vi "AIT 1553 - Parse Tree Messages.vi"(5 "FIFO Idx Qs":T10, 6 "Bus Config Info":T2, 7 "Bus Section":T1, 8 "error out":errorcluster, 10 "Message Refs":T11[](array[typedef]) format="%.0x", 11 "Custom Device Ref":T11 format="%.0x") -> (0 "error out":errorcluster, 2 "Msg Names":string[](array[string]), 3 "Message Settings":T4[](array[typedef]) {"Driver Data"."First Word" min=8 max=31; "Driver Data"."Num Bits" min=1 max=32; "Driver Data"."Start Bit" min=8 max=31; "Block Data Refs"."Data Reference" format="%.0x"})   [LabVIEW 2013, in "AIT 1553 Custom Device.lvlib"]
uses:
  AIT 1553 Custom Device.lvlib
  <vilib>/NI Veristand/Custom Device API/Custom Device Item Ref.ctl
  RT Controls/FIFO Idx Qs.ctl
  RT Controls/AIT 1553 - RT Message Settings.ctl
  <vilib>/NI Veristand/Custom Device API/Block Data Reference.ctl
  <vilib>/NI Veristand/Custom Device API/Data Reference.ctl
  RT Controls/AIT 1553 - Driver Data.ctl
  Controls and Global/Start Bit.ctl
  Controls and Global/Number of Bits.ctl
  RT Controls/AIT 1553 - Board Config Info.ctl
  RT Controls/AIT 1553 - Hardware Type.ctl
  RT Controls/AIT 1553 - Bus Section.ctl
  <vilib>/NI Veristand/Custom Device Tools/Custom Device Utility Library/RT Debug String Color Spec.ctl
  RT Controls/Data Ref FGV Command.ctl
  <instrlib>/AIT 1553/Public/AIT 1553 Controls/Xfer Direction.ctl
  <vilib>/NI Veristand/Custom Device API/Data Access Type.ctl
  Controls and Global/Global.vi
  <vilib>/NI Veristand/Custom Device API/Get Item Property (I32).vi
  <vilib>/NI Veristand/Custom Device API/Get Item Property (Double Array).vi
  <vilib>/NI Veristand/Custom Device API/Get Item Property (U32).vi
  <vilib>/NI Veristand/Custom Device API/Get Item Property (Boolean).vi
  <vilib>/NI Veristand/Custom Device Tools/Custom Device Utility Library/NI VeriStand - Search for Item.vi
  <vilib>/NI Veristand/Custom Device Tools/Custom Device Utility Library/NI VeriStand - Search for All Items by GUID.vi
  <vilib>/NI Veristand/Custom Device Tools/Custom Device Utility Library/NI VeriStand - Search for Item by GUID.vi
  Utility/Print NIVS Debug String.vi
  <vilib>/NI Veristand/Custom Device API/Get Item Property (Double).vi
  <vilib>/NI Veristand/Custom Device API/Custom Device API.lvlib
  <instrlib>/AIT 1553/AIT 1553.lvlib
  <vilib>/NI Veristand/Custom Device Tools/Custom Device Utility Library/Custom Device Utility Library.lvlib
panel:
  in  "Channel handle in":u32
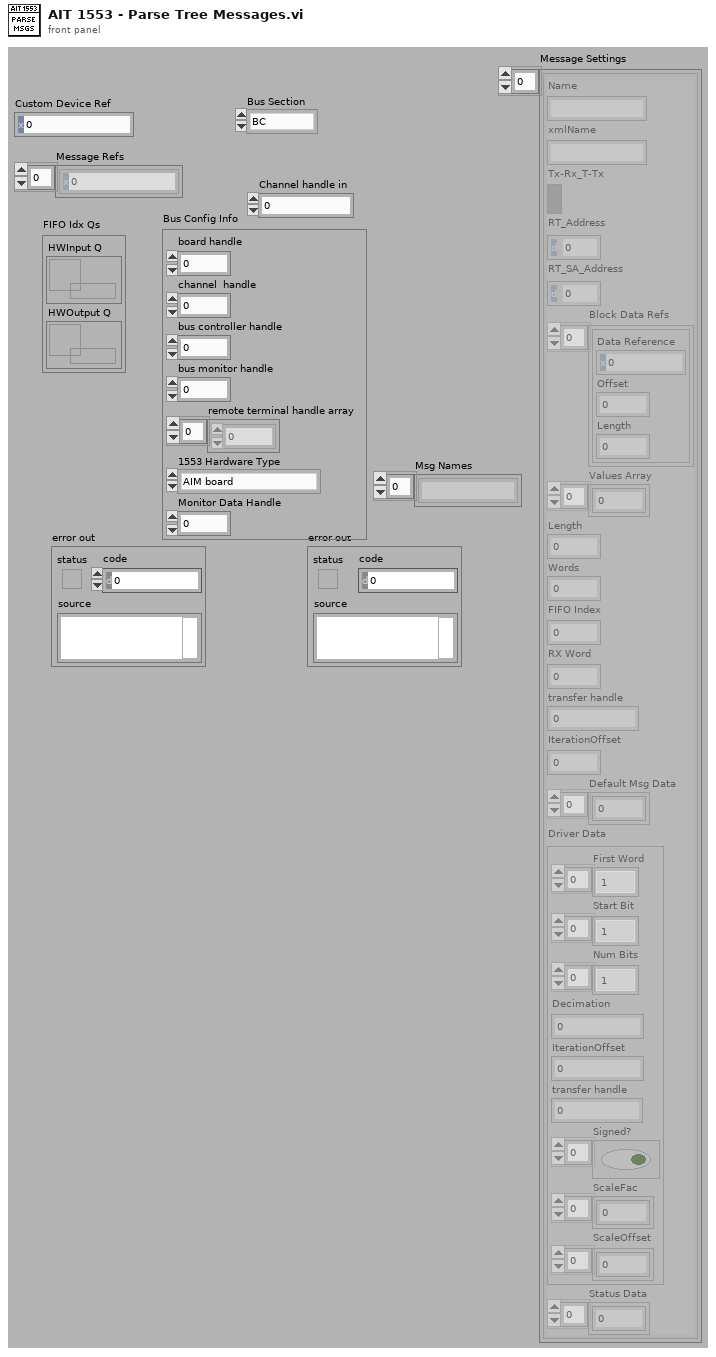
[diagram p1: front panel]
types:
  T1 = typedef "AIT 1553 Custom Device.lvlib/AIT 1553 - Bus Section.ctl" = enum16{"BC", "BM", "RT"}
  T2 = typedef "AIT 1553 Custom Device.lvlib/AIT 1553 - Board Config Info.ctl" = cluster{"board handle":u32, "channel  handle":u32, "bus controller handle":u32, "bus monitor handle":u32, "remote terminal handle array":u32[], "1553 Hardware Type":T3, "Monitor Data Handle":u32}
  T3 = typedef "AIT 1553 Custom Device.lvlib/AIT 1553 - Hardware Type.ctl" = enum16{"AIM board", "AIT Board"}
  T4 = typedef "AIT 1553 Custom Device.lvlib/AIT 1553 - RT Message Settings.ctl" = cluster{"Name":string, "xmlName":string, "Tx-Rx_T-Tx":bool, "RT_Address":u8, "RT_SA_Address":u8, "Block Data Refs":T5[], "Values Array":dbl[], "Length":i32, "Words":i32, "FIFO Index":i32, "RX Word":u32, "transfer handle":u32, "IterationOffset":i32, "Default Msg Data":u16[], "Driver Data":T7, "Status Data":u32[]}
  T5 = typedef "Custom Device API.lvlib/Block Data Reference.ctl" = cluster{"Data Reference":T6, "Offset":i32, "Length":i32}
  T6 = typedef "Custom Device API.lvlib/Data Reference.ctl" = i32
  T7 = typedef "AIT 1553 Custom Device.lvlib/AIT 1553 - Driver Data.ctl" = cluster{"First Word":T8[], "Start Bit":T8[], "Num Bits":T9[], "Decimation":i32, "IterationOffset":i32, "transfer handle":u32, "Signed?":bool[], "ScaleFac":dbl[], "ScaleOffset":dbl[]}
  T8 = typedef "AIT 1553 Custom Device.lvlib/Start Bit.ctl" = i32
  T9 = typedef "AIT 1553 Custom Device.lvlib/Number of Bits.ctl" = i32
  T10 = typedef "AIT 1553 Custom Device.lvlib/FIFO Idx Qs.ctl" = cluster{"HWInput Q":refnum<queue>, "HWOutput Q":refnum<queue>}
  T11 = typedef "Custom Device API.lvlib/Custom Device Item Ref.ctl" = u64
  T12 = typedef "Custom Device Utility Library.lvlib/RT Debug String Color Spec.ctl" = u16
  T13 = typedef "AIT 1553.lvlib/Xfer Direction.ctl" = enum16{"RECEIVE_TRANSFER", "TRANSMIT_TRANSFER"}
  T14 = typedef "AIT 1553 Custom Device.lvlib/Data Ref FGV Command.ctl" = enum16{"Intialize", "Get", "Update"}
  T15 = typedef "Custom Device API.lvlib/Data Access Type.ctl" = enum16{"Read", "Write"}
  T16 = typedef "Custom Device API.lvlib/Custom Device Item Info.ctl" = cluster{"Name":string, "Is Channel":bool, "GUID":string, "Is Waveform":bool}
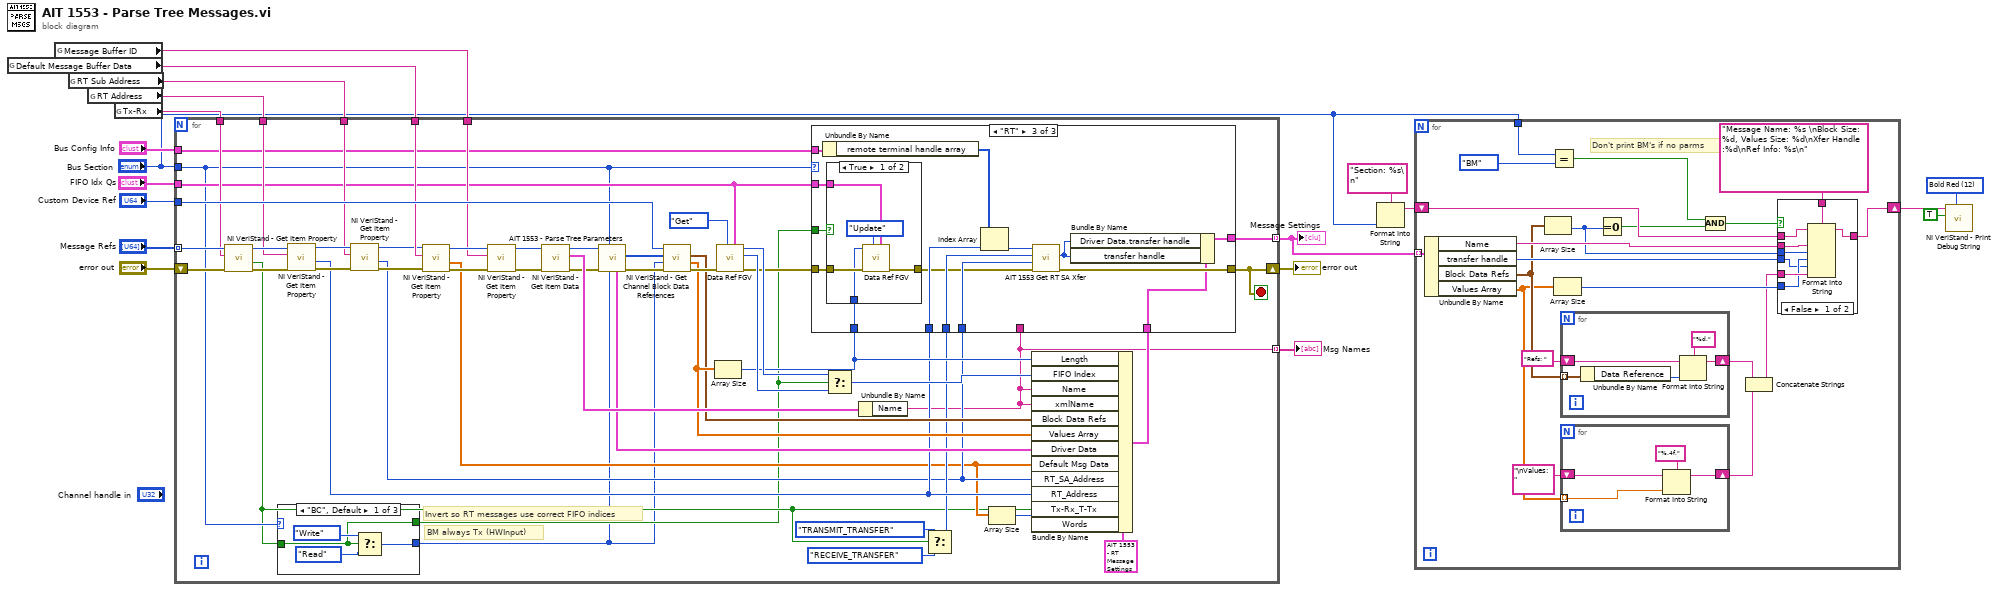
[diagram p0: block diagram]
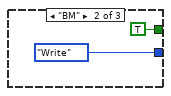
[diagram p3: hidden frame]
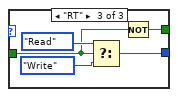
[diagram p4: hidden frame]
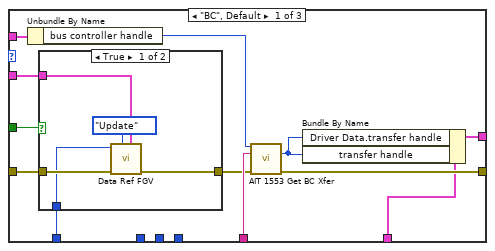
[diagram p5: hidden frame]
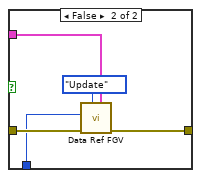
[diagram p6: hidden frame]
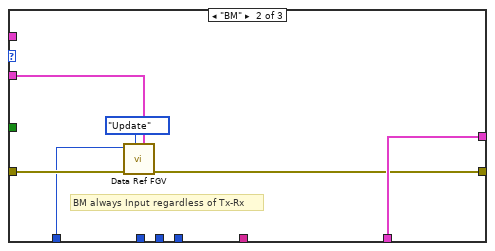
[diagram p7: hidden frame]
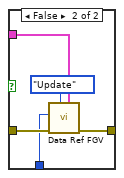
[diagram p8: hidden frame]
diagram:
  w1 = T12 12 items=["Plain White"=7, "Bold White"=15, "Bold Blue"=9, "Bold Green"=10, "Bold Red"=12] ("Attribute")
  n1 = global read "Global.vi" "Default Message Buffer Data"() -> (w11:string)
  n2 = global read "Global.vi" "Message Buffer ID"() -> (w10:string)
  n3 = global read "Global.vi" "RT Sub Address"() -> (w12:string)
  n4 = global read "Global.vi" "RT Address"() -> (w13:string)
  n5 = global read "Global.vi" "Tx-Rx"() -> (w14:string)
  n6 = for {
    tunnel: "Message Refs" -> [w70] mode=indexing
    shift-right: [w60] -> w16
    shift-left: "error out" -> [w61]
    tunnel: "Custom Device Ref" -> [w59]
    tunnel: "FIFO Idx Qs" -> [w33]
    tunnel: w14 -> [w58]
    tunnel: w11 -> [w57]
    tunnel: w13 -> [w52]
    tunnel: w12 -> [w47]
    tunnel: w10 -> [w42]
    tunnel: [w34] -> w4 mode=indexing
    tunnel: "Bus Section" -> [w26]
    tunnel: "Bus Config Info" -> [w32]
    tunnel: [w25] -> w8 mode=indexing
    stop <- w60 stop-if-true
    # "BM always Tx (HWInput)"
    # "Invert so RT messages use correct FIFO indices"
    n7 = call-poly <vilib>:"NI VeriStand - Get Item Property.vi"("error in (no error)"=w61, "Property Name"=w58, "Item Ref in"=w70) -> ("error out"=w53:errorcluster, "Value"=w22:bool, "Item Ref out"=w54:T11)  [unwired: 5 in, 1 out]
    n8 = case shown="\"BC\", Default" w26 {
      tunnel: [w72 Data_Access_Type."Write" ("y") w79] -> w20
      tunnel: w22 -> [w71 _ w78]
      tunnel: [w71 TRUE ("Value") w77] -> w21
      frame "BC", Default {
        n9 = Select(t=Data_Access_Type."Write" ("y"), s=w71, f=Data_Access_Type."Read" ("y")) -> (s? t:f=w72:T15)
      }
      frame "BM" {
      }
      frame "RT" {
        n10 = Select(t=Data_Access_Type."Read" ("y"), s=w78, f=Data_Access_Type."Write" ("y")) -> (s? t:f=w79:T15)
        n11 = Not(x=w78) -> (.not. x?=w77:bool)
      }
    }
    n12 = call-poly <vilib>:"NI VeriStand - Get Item Property.vi"("error in (no error)"=w53, "Property Name"=w52, "Item Ref in"=w54) -> ("error out"=w49:errorcluster, "Value"=w31:i32, "Item Ref out"=w51:T11)  [unwired: 5 in, 1 out]
    n13 = call-poly <vilib>:"NI VeriStand - Get Item Property.vi"("error in (no error)"=w49, "Property Name"=w47, "Item Ref in"=w51) -> ("error out"=w48:errorcluster, "Value"=w27:u32, "Item Ref out"=w50:T11)  [unwired: 5 in, 1 out]
    n14 = call-poly <vilib>:"NI VeriStand - Get Item Property.vi"("error in (no error)"=w48, "Property Name"=w57, "Item Ref in"=w50) -> ("error out"=w44:errorcluster, "Value"=w24:dbl[], "Item Ref out"=w46:T11)  [unwired: 5 in, 1 out]
    n15 = call-poly <vilib>:"NI VeriStand - Get Item Property.vi"("error in (no error)"=w44, "Property Name"=w42, "Item Ref in"=w46) -> ("error out"=w43:errorcluster, "Item Ref out"=w45:T11)  [unwired: 5 in, 2 out]
    n16 = call <vilib>:"NI VeriStand - Get Item Data.vi"("error in (no error)"=w43, "Item Ref in"=w45) -> ("error out"=w56:errorcluster, "Item Info"=w69:T16, "Item Ref out"=w55:T11)  [unwired: 6 in, 1 out]
    n17 = call "AIT 1553 - Parse Tree Parameters.vi"("Access Type"=w20, "Bus Section"=w26, "error in"=w56, "Item Ref in"=w55) -> ("error out"=w67:errorcluster, "Parameter References"=w68:T11[], "Parameter Driver Data"=w38:T7)  [unwired: 4 in, 1 out]
    n18 = call <vilib>:"NI VeriStand - Get Channel Block Data References.vi"("error in (no error)"=w67, "Access"=w20, "Channel Refs"=w68, "Device Ref in"=w59) -> ("error out"=w66:errorcluster, "Values Array"=w40:dbl[], "Block Data Refs"=w39:T5[])  [unwired: 4 in, 1 out]
    n19 = Array Size(array=w40) -> (size(s)=w37:i32)
    n20 = call "Data Ref FGV.vi"("FIFO Idx Qs"=w33, "Command"=Data_Ref_FGV_Command."Get", "error in (no error)"=w66) -> ("error out"=w62:errorcluster, "HWOutput FIFO Index / Length"=w63:i32, "HWInput FIFO Index / Length"=w64:i32)  [unwired: 6 in]
    n21 = Select(t=w64, s=w21, f=w63) -> (s? t:f=w36:i32)
    n22 = Unbundle By Name(w69) -> ("Name"=w25:string)
    n23 = Select(t=Xfer_Direction."TRANSMIT_TRANSFER" ("direction in"), s=w22, f=Xfer_Direction."RECEIVE_TRANSFER" ("direction in")) -> (s? t:f=w28:T13)
    n24 = Array Size(array=w24) -> (size(s)=w23:i32)
    n25 = Bundle By Name(cluster=T4 {"Name"="", "xmlName"="", "Tx-Rx_T-Tx"=FALSE, "RT_Address"=0, "RT_SA_Address"=0, "Block Data Refs"=[], "Values Array"=[], "Length"=0, "Words"=0, "FIFO Index"=0, "RX Word"=0, "transfer handle"=0, "IterationOffset"=0, "Default Msg Data"=[], "Driver Data"={"First Word"=[], "Start Bit"=[], "Num Bits"=[], "Decimation"=0, "IterationOffset"=0, "transfer handle"=0, "Signed?"=[], "ScaleFac"=[], "ScaleOffset"=[]}, "Status Data"=[]} ("Message Settings"), "Length"=w37, "FIFO Index"=w36, "Name"=w25, "xmlName"=w25, "Block Data Refs"=w39, "Values Array"=w40, "Driver Data"=w38, "Default Msg Data"=w24, "RT_SA_Address"=w27, "RT_Address"=w31, "Tx-Rx_T-Tx"=w22, "Words"=w23) -> (w35:T4)
    n26 = case shown="\"RT\"" w26 {
      tunnel: w62 -> [w93 w108 w114]
      tunnel: [w85 w104 w123] -> w60
      tunnel: w37 -> [w92 w106 w112]
      tunnel: w35 -> [w84 w105 w122]
      tunnel: [w83 w105 w121] -> w34
      tunnel: w25 -> [w88 _ _]
      tunnel: w21 -> [w91 _ w115]
      tunnel: w33 -> [w90 w107 w111]
      tunnel: w32 -> [w89 _ w124]
      tunnel: w31 -> [_ _ w120]
      tunnel: w28 -> [_ _ w119]
      tunnel: w27 -> [_ _ w118]
      frame "BC", Default {
        n27 = Unbundle By Name(w89) -> ("bus controller handle"=w87:u32)
        n28 = case shown="True" w91 {
          tunnel: w93 -> [w98 w103]
          tunnel: w92 -> [w96 w101]
          tunnel: w90 -> [w95 w100]
          tunnel: [w94 w99] -> w86
          frame True {
            n29 = call "Data Ref FGV.vi"("FIFO Idx Qs"=w95, "Command"=Data_Ref_FGV_Command."Update", "error in (no error)"=w98, "HWInput Length"=w96) -> ("error out"=w94:errorcluster)  [unwired: 5 in, 2 out]
          }
          frame False {
            n30 = call "Data Ref FGV.vi"("FIFO Idx Qs"=w100, "Command"=Data_Ref_FGV_Command."Update", "error in (no error)"=w103, "HWOutput Length"=w101) -> ("error out"=w99:errorcluster)  [unwired: 5 in, 2 out]
          }
        }
        n31 = call <instrlib>:"AIT 1553 Get BC Xfer.vi"("bus controller handle in"=w87, "transfer description"=w88, "error in"=w86) -> ("transfer handle out"=w82:u32, "error out"=w85:errorcluster)  [unwired: 10 in, 1 out]
        n32 = Bundle By Name(cluster=w84, "Driver Data.transfer handle"=w82, "transfer handle"=w82) -> (w83:T4)
      }
      frame "BM" {
        # "BM always Input regardless of Tx-Rx"
        n33 = call "Data Ref FGV.vi"("FIFO Idx Qs"=w107, "Command"=Data_Ref_FGV_Command."Update", "error in (no error)"=w108, "HWInput Length"=w106) -> ("error out"=w104:errorcluster)  [unwired: 5 in, 2 out]
      }
      frame "RT" {
        n34 = Unbundle By Name(w124) -> ("remote terminal handle array"=w116:u32[])
        n35 = case shown="True" w115 {
          tunnel: w114 -> [w129 w134]
          tunnel: [w127 w131] -> w113
          tunnel: w112 -> [w125 w130]
          tunnel: w111 -> [w126 w132]
          frame True {
            n36 = call "Data Ref FGV.vi"("FIFO Idx Qs"=w126, "Command"=Data_Ref_FGV_Command."Update", "error in (no error)"=w129, "HWInput Length"=w125) -> ("error out"=w127:errorcluster)  [unwired: 5 in, 2 out]
          }
          frame False {
            n37 = call "Data Ref FGV.vi"("FIFO Idx Qs"=w132, "Command"=Data_Ref_FGV_Command."Update", "error in (no error)"=w134, "HWOutput Length"=w130) -> ("error out"=w131:errorcluster)  [unwired: 5 in, 2 out]
          }
        }
        n38 = Index Array(array=w116, index=w120) -> (element=w117:u32)
        n39 = call <instrlib>:"AIT 1553 Get RT SA Xfer.vi"("error in"=w113, "subaddress in"=w118, "direction in"=w119, "remote terminal handle in"=w117) -> ("error out"=w123:errorcluster, "transfer handle out"=w110:u32)  [unwired: 5 in, 1 out]
        n40 = Bundle By Name(cluster=w122, "Driver Data.transfer handle"=w110, "transfer handle"=w110) -> (w121:T4)
      }
    }
  }
  "error out" <- w16
  "Message Settings" <- w4
  "Msg Names" <- w8
  n41 = Format Into String(format string="Section: %s\n", "Bus Section") -> (resulting string=w7:string)  [unwired: 2 in, 1 out]
  n42 = for {
    tunnel: w4 -> [w154] mode=indexing
    shift-right: [w149] -> w3
    shift-left: w7 -> [w150]
    tunnel: "Bus Section" -> [w147]
    # "Don't print BM's if no parms"
    n43 = Unbundle By Name(w154) -> ("Name"=w152:string, "transfer handle"=w151:u32, "Block Data Refs"=w145:T5[], "Values Array"=w138:dbl[])
    n44 = Array Size(array=w145) -> (size(s)=w141:i32)
    n45 = Equal?(x=w147, y=AIT_1553_-_Bus_Section."BM") -> (x = y?=w142:bool)
    n46 = Array Size(array=w138) -> (size(s)=w140:i32)
    n47 = for {
      tunnel: w145 -> [w172] mode=indexing
      shift-right: [w169] -> w137
      shift-left: "Refs: " ("format string") -> [w170]
      n48 = Unbundle By Name(w172) -> ("Data Reference"=w168:T6)
      n49 = Format Into String(format string="%d,", initial string=w170, w168) -> (resulting string=w169:string)  [unwired: 1 in, 1 out]
    }
    n50 = for {
      tunnel: w138 -> [w155] mode=indexing
      shift-right: [w156] -> w136
      shift-left: "\nValues: " ("format string") -> [w157]
      n51 = Format Into String(format string="%.4f,", initial string=w157, w155) -> (resulting string=w156:string)  [unwired: 1 in, 1 out]
    }
    n52 = Equal To 0?(x=w141) -> (x = 0?=w143:bool)
    n53 = Compound Arithmetic op=AND(w142, w143) -> (w144:bool)
    n54 = Concatenate Strings(w137, w136) -> (w135:string)
    n55 = case shown="False" w144 {
      tunnel: "Message Name: %s \nBlock Size: %d, Values Size: %d\nXfer Handle :%d\nRef Info: %s\n" ("format string") -> [w166 _]
      tunnel: w152 -> [w162 _]
      tunnel: w151 -> [w159 _]
      tunnel: w150 -> [w165 w167]
      tunnel: [w164 w167] -> w149
      tunnel: w135 -> [w163 _]
      tunnel: w141 -> [w161 _]
      tunnel: w140 -> [w160 _]
      frame False {
        n56 = Format Into String(format string=w166, initial string=w165, w162, w161, w160, w159, w163) -> (resulting string=w164:string)  [unwired: 1 in, 1 out]
      }
      frame True {
      }
    }
  }
  n57 = call <vilib>:"NI VeriStand - Print Debug String.vi"("Attribute"=w1, "Add to log file? (T)"=TRUE, "Message"=w3) -> ()  [unwired: 8 in, 1 out]
